vi "Write Local Resource.vi"(8 "error in (no error)":errorcluster, 10 "Local Resource":refnum<visa-resource-name>, 11 "57XX in":refnum<class "57XX.lvclass">) -> (0 "error out":errorcluster, 3 "57XX out":refnum<class "57XX.lvclass">)   [LabVIEW 2019, in "57XX.lvlib" / "57XX.lvclass"]
uses:
  Library/57XX.lvclass
  Library/57XX.lvclass/57XX.ctl
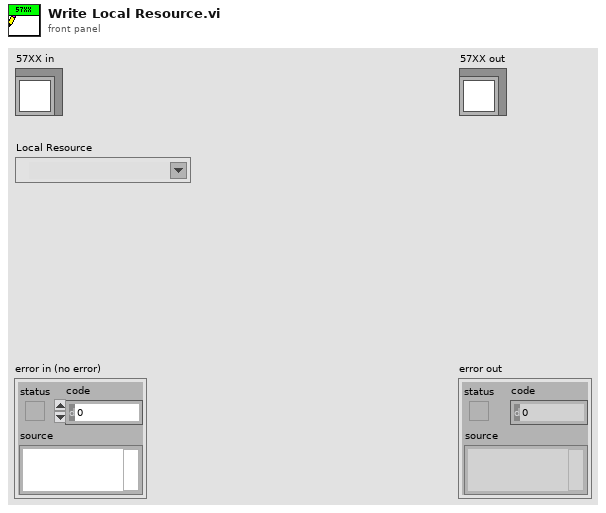
[diagram p1: front panel]
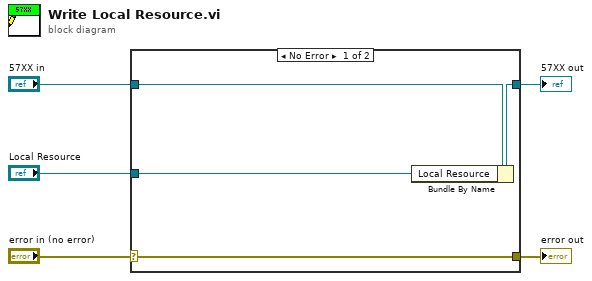
[diagram p0: block diagram]
diagram:
  n1 = case shown="No Error" "error in (no error)" {
    selector: "error in (no error)" -> [w9 w10]
    tunnel: [w9 w10] -> w4
    tunnel: [w7 w11] -> w2
    tunnel: "57XX in" -> [w8 w11]
    tunnel: "Local Resource" -> [w6 _]
    frame No Error {
      n2 = Bundle By Name(cluster=w8, "Local Resource"=w6) -> (w7:refnum<class "57XX.lvclass">)
    }
    frame Error {
    }
  }
  "error out" <- w4
  "57XX out" <- w2
